vi "Power Output Format Plot.vi"(6 "Measured Values":refnum<vi>, 8 "error in (no error)":errorcluster, 9 "Reset Plot? (F)":bool, 10 "Test Parameters":T1={"Stimulus"={"Frequency Type"=enum."Band Edges", "Frequency Ranges"=[], "TX 1 Frequency (MHz)"={"Min"=0.0, "Max"=0.0}, "TX 2 Frequency (MHz)"={"Min"=0.0, "Max"=0.0}, "RX Frequency (MHz)"={"Min"=0.0, "Max"=0.0}, "Pad Model Number"="", "Pad Serial Number"="", "Pad Values"=[]}, "Measurement"={"DUT Port"=enum."Port 1", "Direction"=0, "Frequency Step Size"=0}, "Display"={"Frequency"={"Min"=-1.0, "Max"=-1.0}, "Power"={"Min"=-1, "Max"=-1}}, "Limit"={"Min Power (dBm)"=44.0}, "Calibration"={"Calibrated?"=FALSE}} {"Measurement"."Frequency Step Size" items=["0.2", "0.4", "1.0", "2.0", "4.0"]; "Measurement"."Direction" items=["Reverse", "Forward", "Auxiliary"]}, 11 "Plots":T10) -> (0 "error out":errorcluster)   [LabVIEW 2011]
uses:
  TypeDefs/Power Output Test Parameters.ctl
  TypeDefs/Power Output Stimulus Parameters.ctl
  TypeDefs/Power Output Measurement Parameters.ctl
  BPIMCore EXT/HW IO/DUTport.ctl
  BPIMCore EXT/HW IO/MeasMode.ctl
  BPIMCore EXT/HW IO/PIM Sweep Step Size.ctl
  TypeDefs/Power Output Display Parameters.ctl
  TypeDefs/Power Output Limit Parameters.ctl
  TypeDefs/Power Output Calibration State.ctl
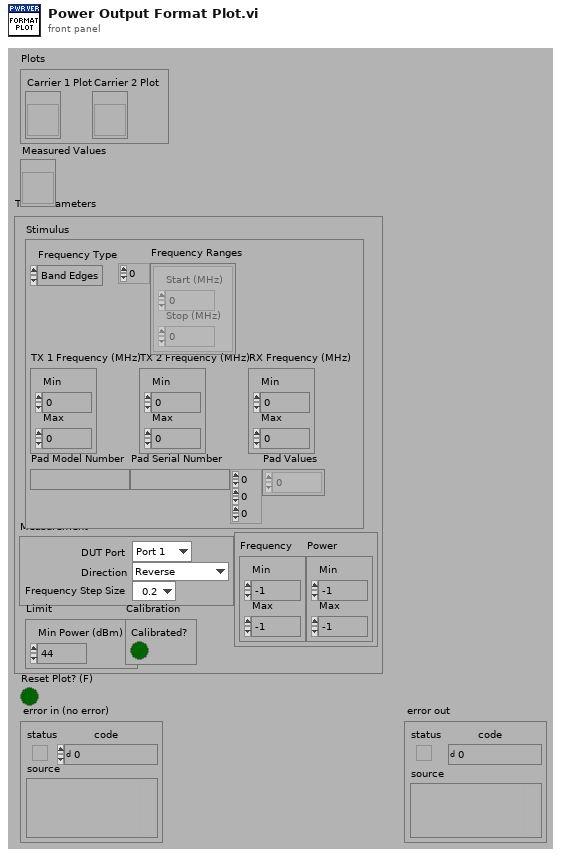
[diagram p1: front panel]
types:
  T1 = typedef "Power Output Test Parameters.ctl" = cluster{"Stimulus":T2, "Measurement":T3, "Display":T7, "Limit":T8, "Calibration":T9}
  T2 = typedef "Power Output Stimulus Parameters.ctl" = cluster{"Frequency Type":enum16{"Band Edges", "Custom"}, "Frequency Ranges":cluster{"Start (MHz)":dbl, "Stop (MHz)":dbl}[], "TX 1 Frequency (MHz)":cluster{"Min":dbl, "Max":dbl}, "TX 2 Frequency (MHz)":cluster{"Min":dbl, "Max":dbl}, "RX Frequency (MHz)":cluster{"Min":dbl, "Max":dbl}, "Pad Model Number":string, "Pad Serial Number":string, "Pad Values":dbl[][][]}
  T3 = typedef "Power Output Measurement Parameters.ctl" = cluster{"DUT Port":T4, "Direction":T5, "Frequency Step Size":T6}
  T4 = typedef "DUTport.ctl" = enum16{"Port 1", "Port 2"}
  T5 = typedef "MeasMode.ctl" = u16
  T6 = typedef "PIM Sweep Step Size.ctl" = u16
  T7 = typedef "Power Output Display Parameters.ctl" = cluster{"Frequency":cluster{"Min":dbl, "Max":dbl}, "Power":cluster{"Min":i32, "Max":i32}}
  T8 = typedef "Power Output Limit Parameters.ctl" = cluster{"Min Power (dBm)":dbl}
  T9 = typedef "Power Output Calibration State.ctl" = cluster{"Calibrated?":bool}
  T10 = cluster{"Carrier 1 Plot":refnum<vi>, "Carrier 2 Plot":refnum<vi>}
  T11 = cluster{"Array Constant":dbl[], "Array Constant":dbl[]}[]
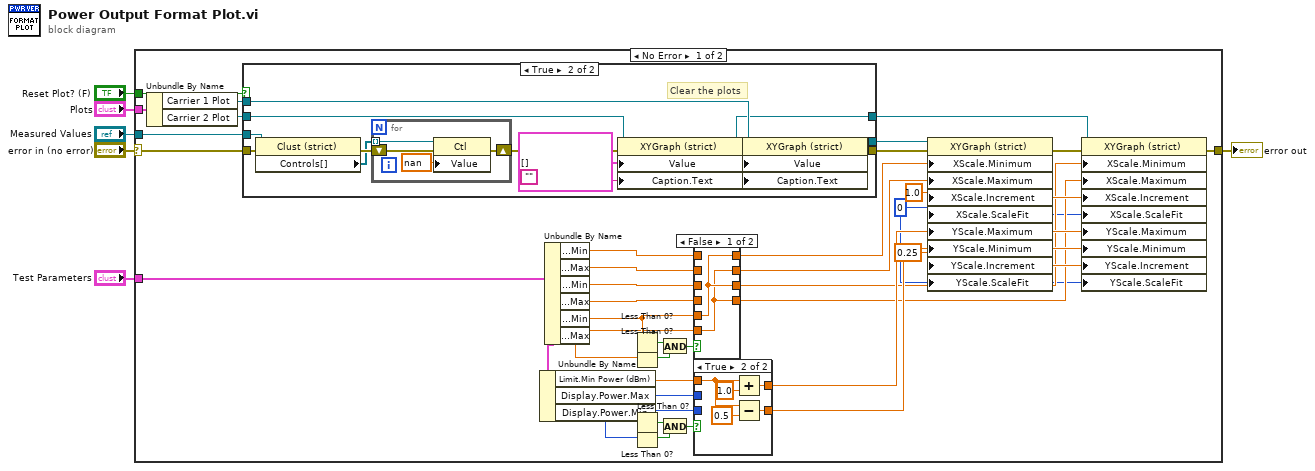
[diagram p0: block diagram]
diagram:
  n1 = case shown="No Error" "error in (no error)" {
    selector: "error in (no error)" -> [w42 w76]
    tunnel: "Reset Plot? (F)" -> [w41 _]
    tunnel: [w19 w76] -> w5
    tunnel: "Plots" -> [w38 _]
    tunnel: "Test Parameters" -> [w22 _]
    tunnel: "Measured Values" -> [w12 _]
    frame No Error {
      w13 = 0.25 ("Y Scale.Range:Increment")
      w7 = u8 0 ("X Scale.Scale Fit")
      w14 = 1.0 ("X Scale.Range:Increment")
      n2 = Unbundle By Name(w38) -> ("Carrier 1 Plot"=w37:refnum<vi>, "Carrier 2 Plot"=w36:refnum<vi>)
      n3 = case shown="True" w41 {
        tunnel: w42 -> [w57 w62]
        tunnel: w37 -> [w58 w71]
        tunnel: [w57 w70] -> w39
        tunnel: [w58 w69] -> w40
        tunnel: w36 -> [w56 w68]
        tunnel: [w56 w67] -> w20
        tunnel: w12 -> [_ w59]
        frame False {
        }
        frame True {
          w64 = ""
          w65 = T11 [] ("Value")
          # "Clear the plots"
          n4 = property class="Clust (strict)"(reference=w59, error in=w62) -> (error out=w61:errorcluster, "Controls[]"=w60:refnum<vi>[])  [unwired: 1 out]
          n5 = for {
            shift-right: [w74] -> w63
            shift-left: w61 -> [w75]
            tunnel: w60 -> [w73] mode=indexing
            n6 = property class="Ctl"(reference=w73, error in=w75, "Value"=nan) -> (error out=w74:errorcluster)  [unwired: 1 out]
          }
          n7 = property class="XYGraph (strict)"(reference=w68, error in=w63, "Value"=w65, "Caption.Text"=w64) -> (reference out=w67:refnum<vi>, error out=w66:errorcluster)
          n8 = property class="XYGraph (strict)"(reference=w71, error in=w66, "Value"=w65, "Caption.Text"=w64) -> (reference out=w69:refnum<vi>, error out=w70:errorcluster)
        }
      }
      n9 = Unbundle By Name(w22) -> ("Limit.Min Power (dBm)"=w26:dbl, "Display.Power.Max"=w27:i32, "Display.Power.Min"=w28:i32)
      n10 = Unbundle By Name(w22) -> ("Stimulus.TX 1 Frequency (MHz).Min"=w32:dbl, "Stimulus.TX 1 Frequency (MHz).Max"=w31:dbl, "Stimulus.TX 2 Frequency (MHz).Min"=w11:dbl, "Stimulus.TX 2 Frequency (MHz).Max"=w10:dbl, "Display.Frequency.Min"=w30:dbl, "Display.Frequency.Max"=w29:dbl)
      n11 = Less Than 0?(x=w30) -> (x < 0?=w35:bool)
      n12 = Less Than 0?(x=w29) -> (x < 0?=w34:bool)
      n13 = Less Than 0?(x=w27) -> (x < 0?=w23:bool)
      n14 = Less Than 0?(x=w28) -> (x < 0?=w24:bool)
      n15 = And(x=w35, y=w34) -> (x .and. y?=w33:bool)
      n16 = And(x=w23, y=w24) -> (x .and. y?=w25:bool)
      n17 = case shown="False" w33 {
        tunnel: w32 -> [_ w55]
        tunnel: w31 -> [_ w54]
        tunnel: [w51 w55] -> w18
        tunnel: [w50 w54] -> w17
        tunnel: w30 -> [w51 _]
        tunnel: w29 -> [w50 _]
        tunnel: [w51 w53] -> w9
        tunnel: w11 -> [_ w53]
        tunnel: [w50 w52] -> w8
        tunnel: w10 -> [_ w52]
        frame False {
        }
        frame True {
        }
      }
      n18 = case shown="True" w25 {
        tunnel: w26 -> [_ w46]
        tunnel: [w44 w49] -> w16
        tunnel: [w43 w48] -> w15
        tunnel: w27 -> [w44 _]
        tunnel: w28 -> [w43 _]
        frame False {
        }
        frame True {
          n19 = Add(x=w46, y=1.0) -> (x+y=w49:dbl)
          n20 = Subtract(x=w46, y=0.5) -> (x-y=w48:dbl)
        }
      }
      n21 = property class="XYGraph (strict)"(reference=w40, error in=w39, "XScale.Minimum"=w18, "XScale.Maximum"=w17, "XScale.Increment"=w14, "XScale.ScaleFit"=w7, "YScale.Maximum"=w16, "YScale.Minimum"=w15, "YScale.Increment"=w13, "YScale.ScaleFit"=w7) -> (error out=w21:errorcluster)  [unwired: 1 out]
      n22 = property class="XYGraph (strict)"(reference=w20, error in=w21, "XScale.Minimum"=w9, "XScale.Maximum"=w8, "XScale.Increment"=w14, "XScale.ScaleFit"=w7, "YScale.Maximum"=w16, "YScale.Minimum"=w15, "YScale.Increment"=w13, "YScale.ScaleFit"=w7) -> (error out=w19:errorcluster)  [unwired: 1 out]
    }
    frame Error {
    }
  }
  "error out" <- w5
